vi "Process.vi"(8 "error in":errorcluster, 11 "main_UI":refnum<class "UI_main.lvclass">) -> (0 "error out":errorcluster, 3 "main_UI out":refnum<class "UI_main.lvclass">)   [LabVIEW 2016, in "UI_main.lvclass"]
doc: "---------------------------------------------------------------\nJKI State Machine Objects™\nhttp://jki.net/state-machine-objects/\nCopyright (C) 2005-2015, JKI <info@jki.net>\nALL RIGHTS RESERVED"
uses:
  UI_main.lvclass
  C:/Program Files (x86)/National Instruments/LabVIEW 2016/vi.lib/JKI/JKI SMO/SMO/SMO.lvclass
  <vilib>/JKI/JKI SMO/SMO/Typedefs/Parent Call--Enum.ctl
  SMO.Activity/SMO.Activity.lvclass
  <vilib>/JKI/JKI SMO/SMO/SMO.lvclass
  DAQ_config_UI/UI_DAQ_config.lvclass
  C:/user/patrick/hg/lockin.SMO/lvsrc/SMOs/SMO.Activity/SMO.Activity.lvclass
panel:
  in  "Shutdown":bool
  in  "config Lockin":bool
  in  "config DAQs":bool
  in  "show graphs":bool
  # "For instructions on how to use the JKI State Machine Objects, examples and video tutorials, visit:\nhttp://jki.net/state-machine-objects/\n\nJKI State Machine Objects™\nhttp://jki.net/state-machine-objects/\nCopyright (C) 2005-2015, JKI <info@jki.net>\nALL RIGHTS RESERVED"
  # "main UI: Always running?"
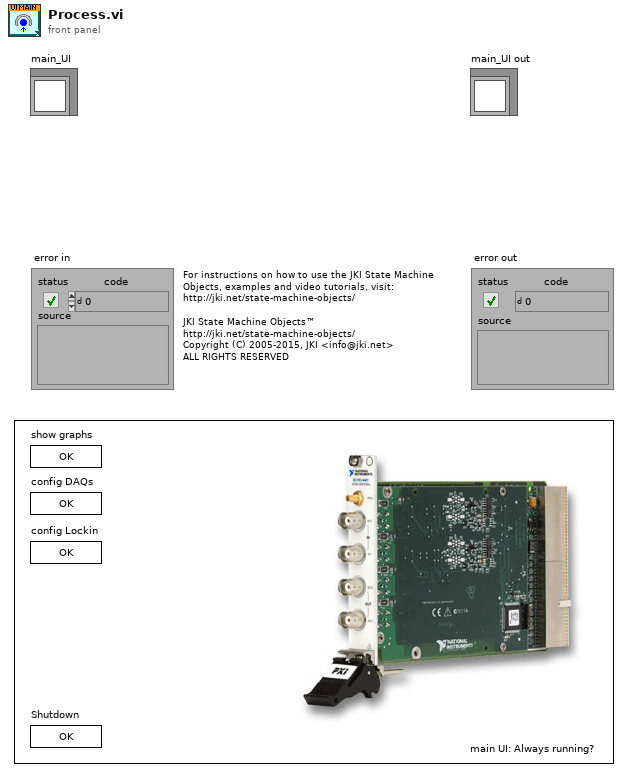
[diagram p1: front panel]
types:
  T1 = typedef "SMO.lvclass/Parent Call--Enum.ctl" = enum16{"Allows parent to run", "Does not request parent to run"}
  T2 = enum32{"invalid app kind", "Development System", "Run Time System", "Student Edition", "Embedded LabVIEW", "Evaluation", "Custom"}
  T3 = enum32{"Invalid", "Standard", "Closed", "Hidden", "Minimized", "Maximized"}
  T4 = enum32{"Bad", "Idle", "Run top level", "Running"}
  T5 = cluster{"Core":cluster{"Current VI Reference":refnum<vi>, "Close Panel on Exit?":bool, "error":errorcluster}, "Self Reference":refnum<class "UI_main.lvclass">, "Your string data":string, "SubUIs":refnum<class "SMO.Activity.lvclass">[]}
  T6 = cluster{"Current VI Reference":refnum<vi>, "Close Panel on Exit?":bool, "error":errorcluster}
  T7 = typedef "SMO.lvclass/Protected Events.ctl" = cluster{"StopProcesses":refnum<user-event>, "AbortProcesses":refnum<user-event>, "Config Changed":refnum<user-event>, "Dependency":refnum<user-event>}
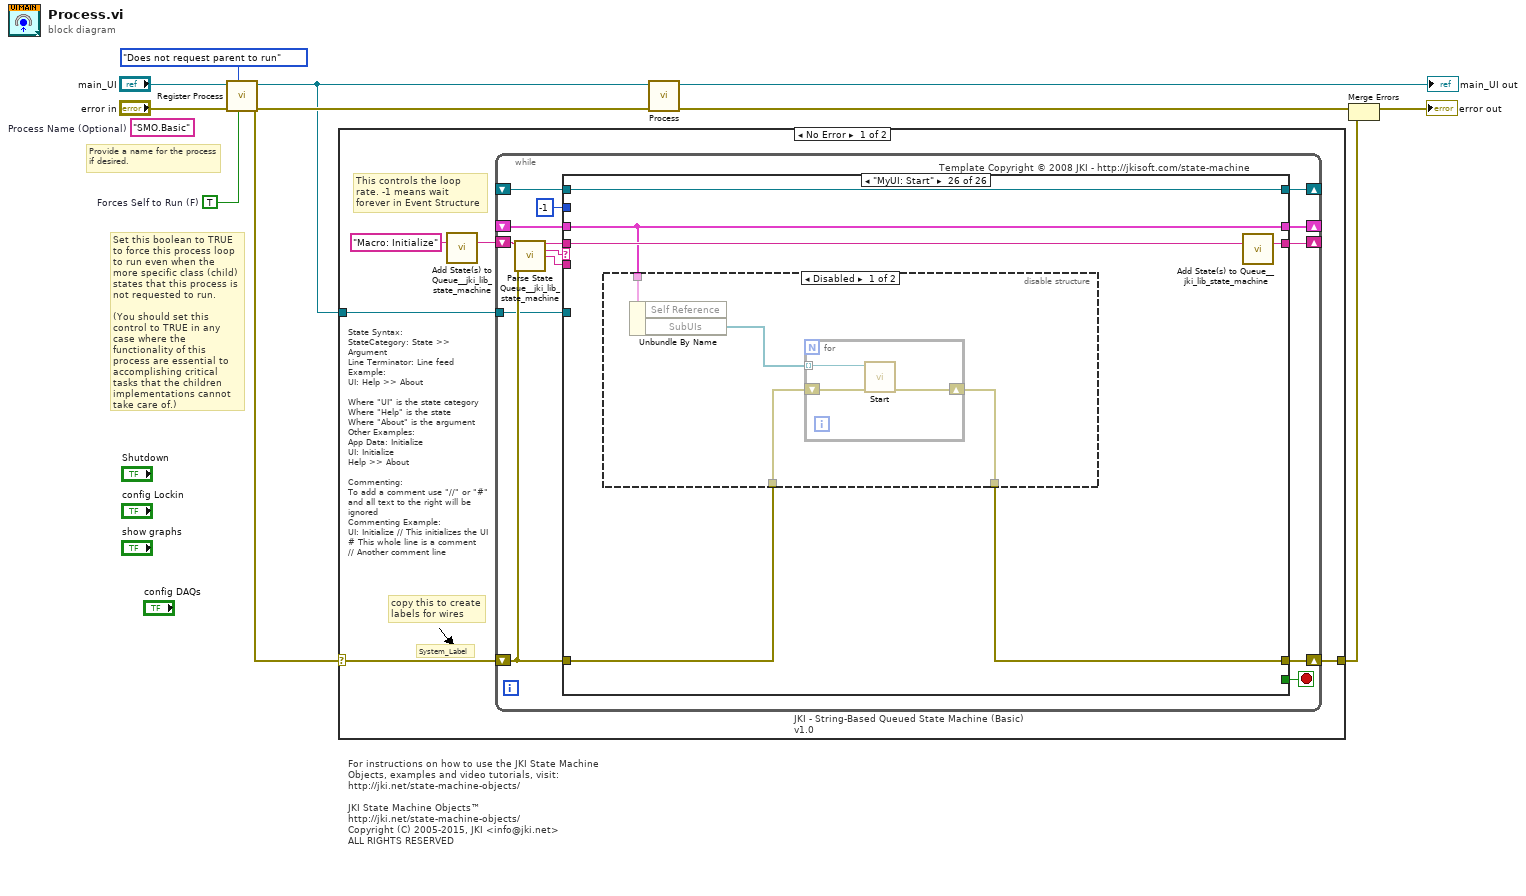
[diagram p0: block diagram]
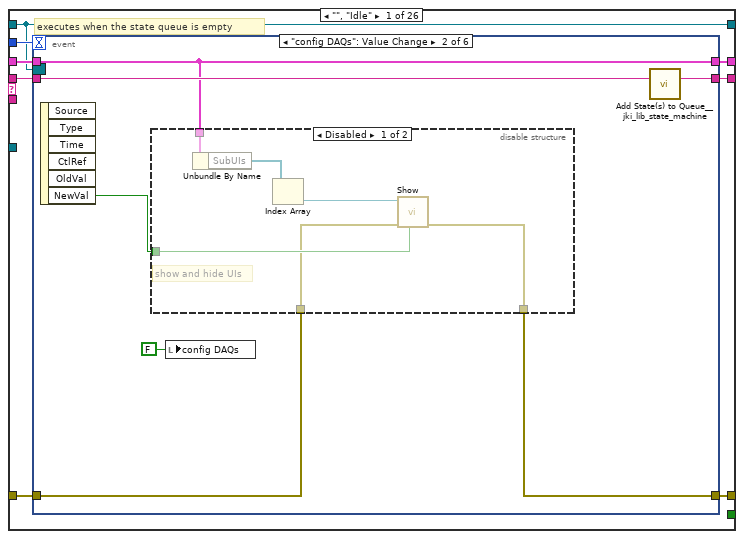
[diagram p2: hidden frame]
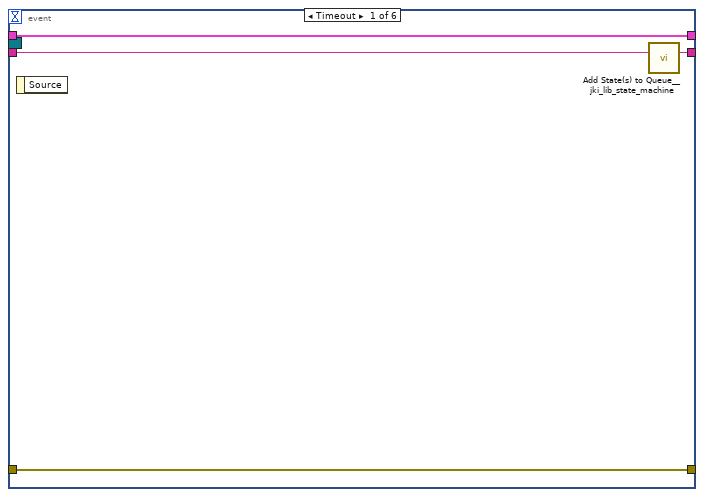
[diagram p3: hidden frame]
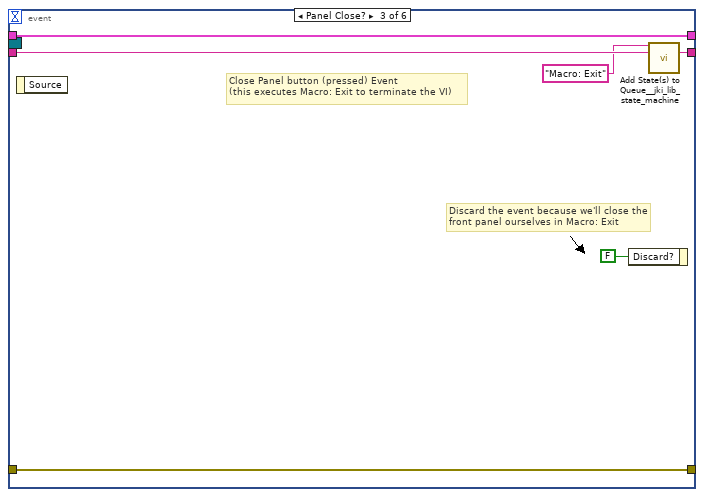
[diagram p5: hidden frame]
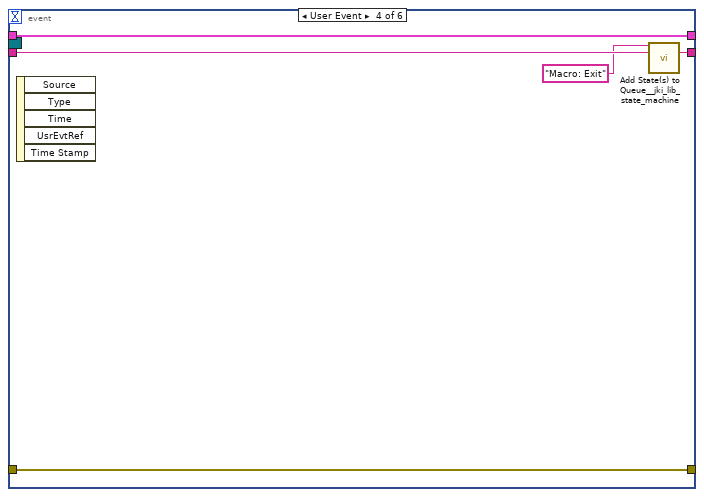
[diagram p6: hidden frame]
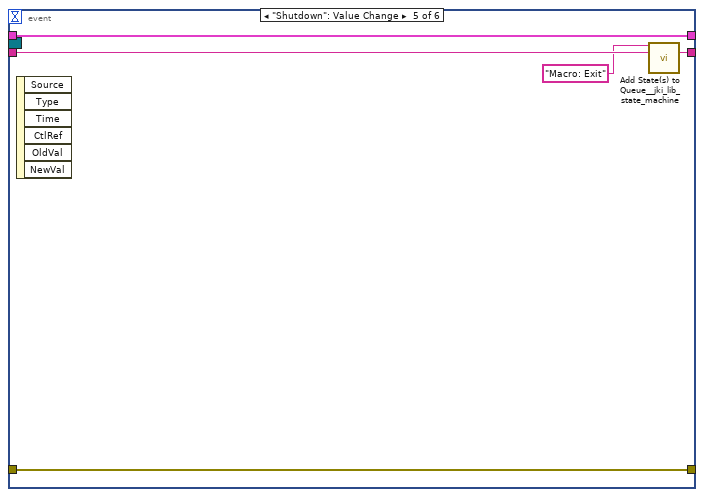
[diagram p7: hidden frame]
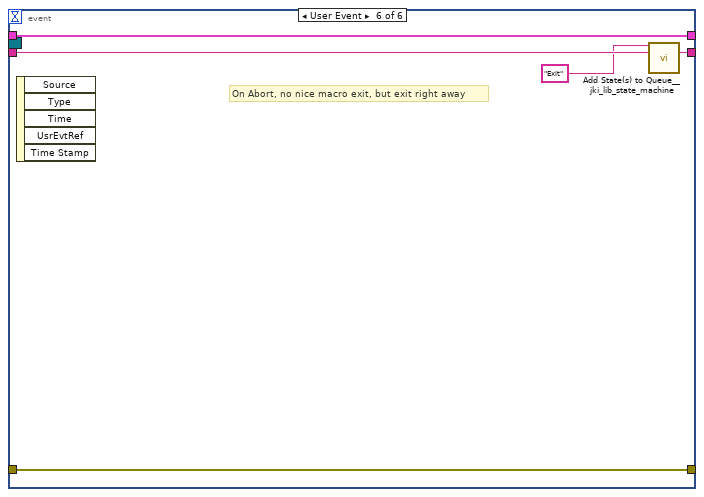
[diagram p8: hidden frame]
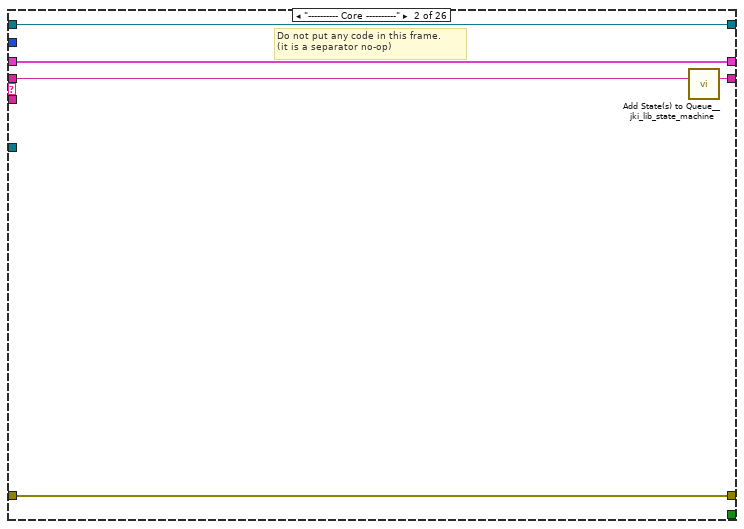
[diagram p9: hidden frame]
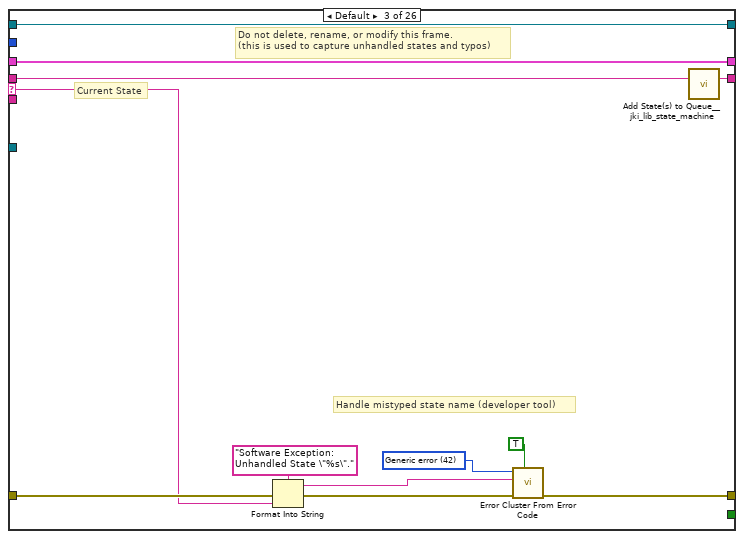
[diagram p10: hidden frame]
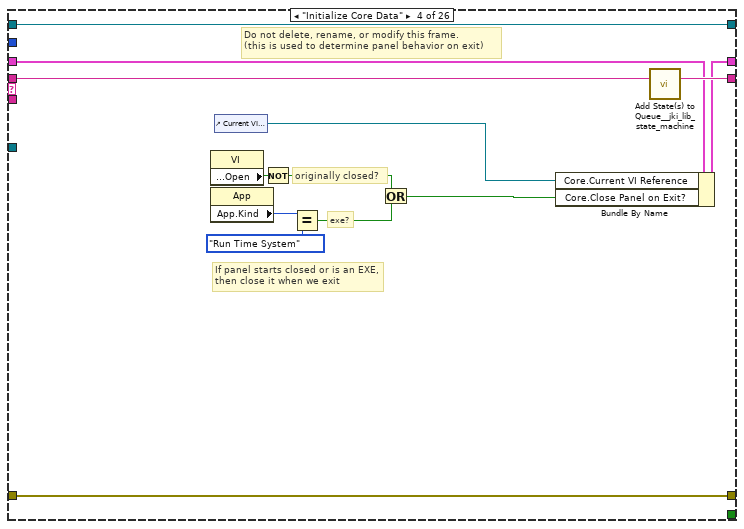
[diagram p11: hidden frame]
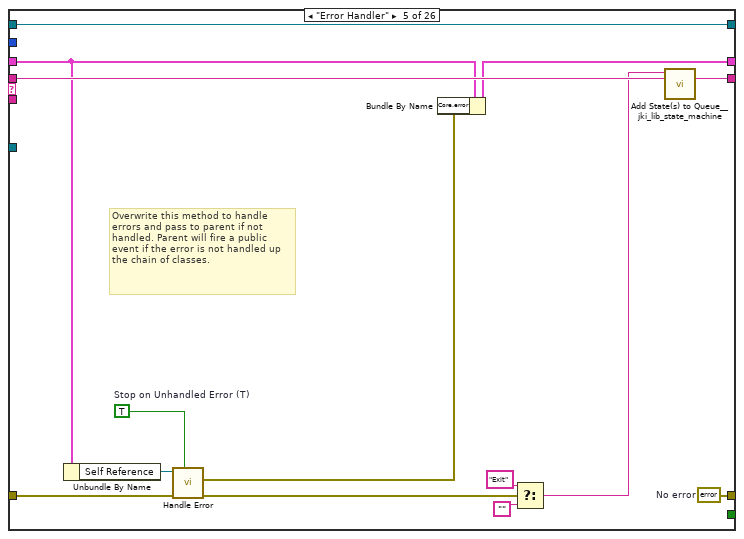
[diagram p12: hidden frame]
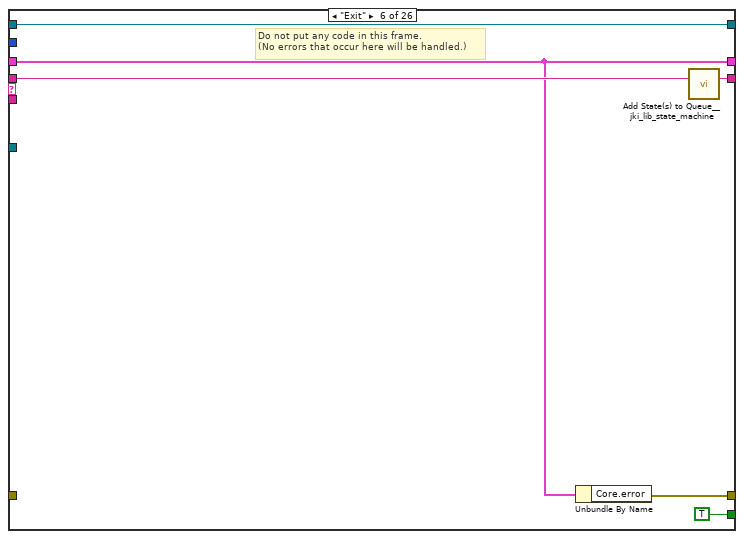
[diagram p13: hidden frame]
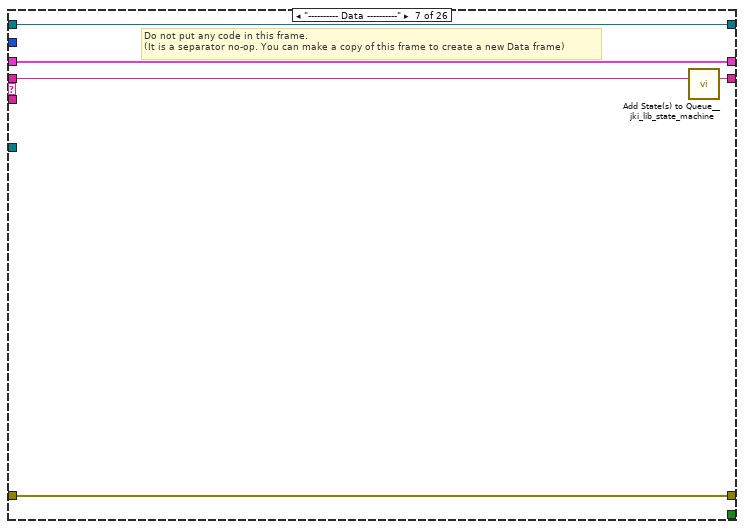
[diagram p14: hidden frame]
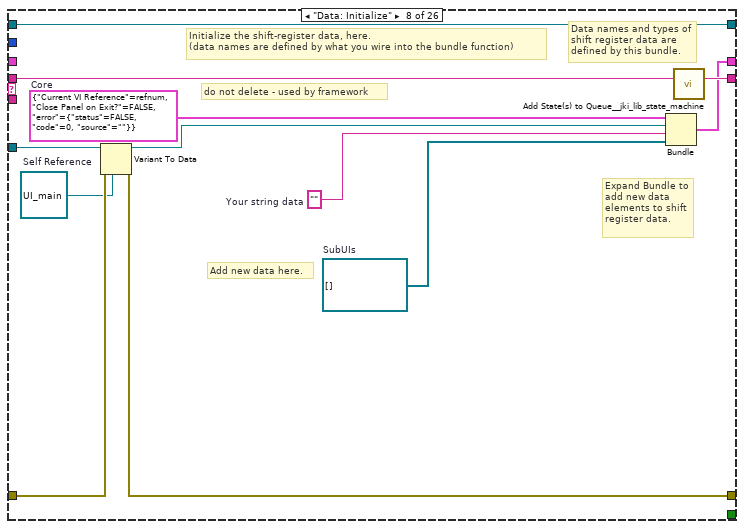
[diagram p15: hidden frame]
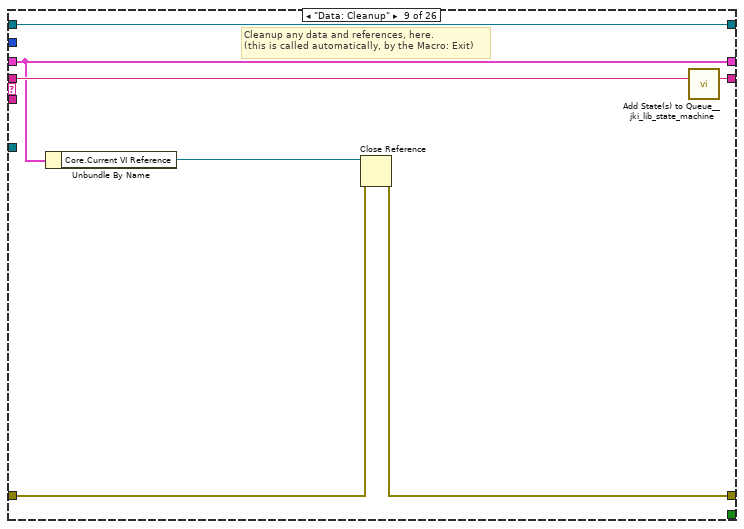
[diagram p16: hidden frame]
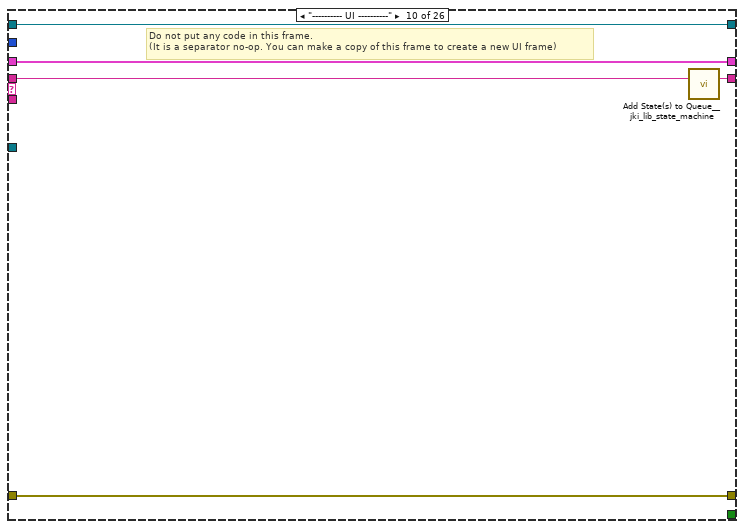
[diagram p17: hidden frame]
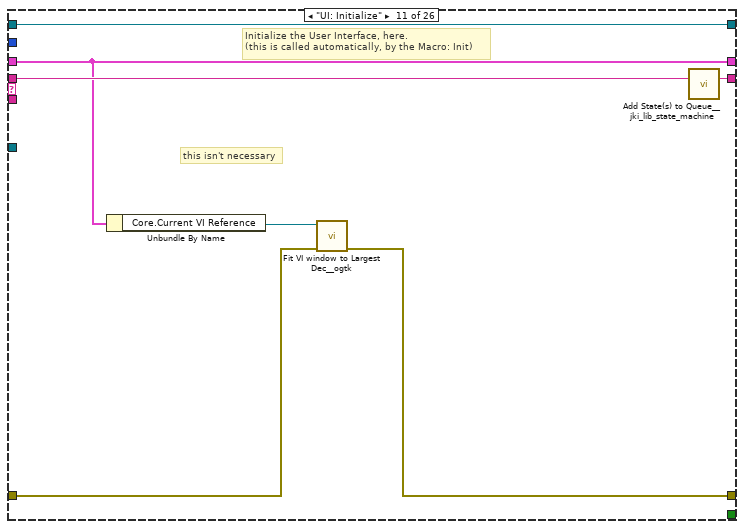
[diagram p18: hidden frame]
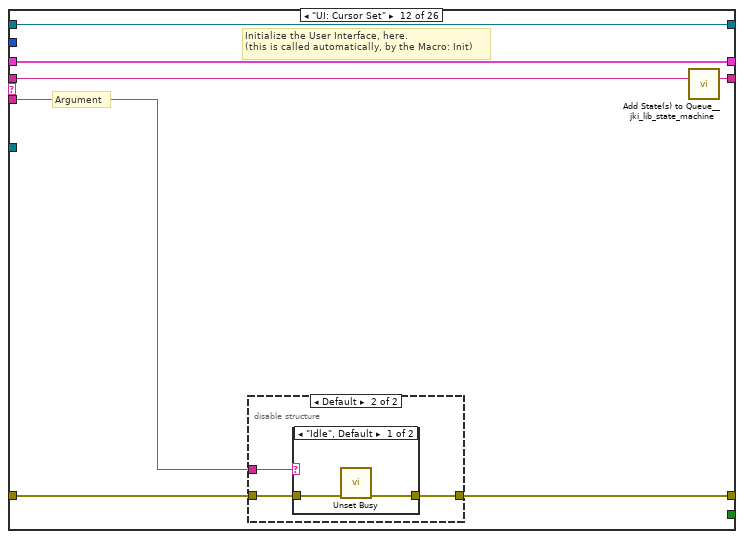
[diagram p19: hidden frame]
diagram:
  w1 = TRUE  # Forces Self to Run (F)
  (unwired) "SMO.Basic"  # Process Name (Optional)
  # "Provide a name for the process\nif desired."
  # "Set this boolean to TRUE to force this process loop to run even when the more specific class (child) states that this process is not requested to run.\n\n(You should set this control to TRUE in any case where the functionality of this process are essential to accomplishing critical tasks that the children implementations cannot take care of.)"
  # "For instructions on how to use the JKI State Machine Objects, examples and video tutorials, visit:\nhttp://jki.net/state-machine-objects/\n\nJKI State Machine Objects™\nhttp://jki.net/state-machine-objects/\nCopyright (C) 2005-2015, JKI <info@jki.net>\nALL RIGHTS RESERVED"
  n1 = call <vilib>:"Register Process.vi"("Forces Self to Run (F)"=w1, "Parent Call"=Parent_Call--Enum."Does not request parent to run", "error in (no error)"="error in", "SMO"="main_UI") -> ("error out"=w7:errorcluster, "SMO out"=w6:refnum<class "UI_main.lvclass">)  [unwired: 6 in]
  n2 = case shown="No Error" w7 {
    selector: w7 -> [w12 w354]
    tunnel: w6 -> [w13 _]
    tunnel: [w11 w354] -> w3
    frame No Error {
      # "State Syntax:\nStateCategory: State >> Argument\nLine Terminator: Line feed\nExample:\nUI: Help >> About\n\nWhere \"UI\" is the state category\nWhere \"Help\" is the state\nWhere \"About\" is the argument\nOther Examples:\nApp Data: Initialize\nUI: Initialize\nHelp >> About\n\nCommenting:\nTo add a comment use \"//\" or \"#\" and all text to the right will be ignored\nCommenting Example:\nUI: Initialize // This initializes the UI\n# This whole line is a comment\n// Another comment line"
      # "copy this to create labels for wires"
      # "This controls the loop rate. -1 means wait forever in Event Structure"
      # "System_Label"
      n3 = call <vilib>:"Add State(s) to Queue__jki_lib_state_machine.vi"("State(s) in (\"\")"="Macro: Initialize") -> ("States Out"=w15:string)  [unwired: 14 in]
      n4 = while "JKI - String-Based Queued State Machine (Basic) v1.0" {
        shift-right: [w22] -> _
        shift-left: _ -> [w21]
        shift-right: [w25] -> w11
        shift-left: w12 -> [w19]
        shift-right: [w24] -> _
        shift-left: w15 -> [w26]
        tunnel: w13 -> [w18]
        shift-right: [w17] -> _
        shift-left: _ -> [w16]
        stop <- w23 stop-if-true
        # "Template Copyright © 2008 JKI - http://jkisoft.com/state-machine"
        n5 = call <vilib>:"Parse State Queue__jki_lib_state_machine.vi"("State Queue"=w26, "Error In (no error)"=w19) -> ("Remaining States"=w28:string, "Current State"=w29:string, "Arguments"=w27:string)  [unwired: 11 in]
        n6 = case shown="\"MyUI: Start\"" w29 {
          selector: w29 -> [_ _ w82 _ _ _ _ _ _ _ _ _ _ _ _ _ _ _ _ _ _ _ _ _ _ _]
          tunnel: w28 -> [w37 w80 w86 w105 w119 w125 w130 w142 w149 w154 w161 w168 w186 w218 w232 w246 w251 w262 w267 w277 w283 w288 w295 w320 w333 w346]
          tunnel: w27 -> [_ _ _ _ _ _ _ _ _ _ _ w162 w181 _ _ _ _ _ _ _ _ _ _ _ _ _]
          tunnel: w21 -> [w35 w77 w84 w96 w113 w121 w127 _ w144 w151 w156 w166 w183 w215 w228 w237 w248 w259 w264 w275 w281 w286 w292 w317 w330 w343]
          tunnel: [w34 w78 w88 w102 w114 w120 w128 w137 w145 w152 w157 w163 w178 w216 w230 w244 w249 w253 w265 w270 w279 w284 w289 w315 w328 w341] -> w25
          tunnel: w19 -> [w33 w78 w87 w102 w115 _ w128 w138 w146 w152 w158 w164 w184 w216 w230 w244 w249 w254 w265 w271 w279 w284 w290 w316 w329 w342]
          tunnel: [w36 w79 w85 w104 w118 w124 w129 w141 w148 w153 w160 w167 w185 w217 w231 w245 w250 w261 w266 w276 w282 w287 w294 w319 w332 w345] -> w24
          tunnel: [_ _ _ _ _ TRUE _ _ _ _ _ _ _ _ _ _ _ _ _ _ _ _ _ _ _ _] -> w23
          tunnel: [w32 w77 w84 w103 w112 w121 w127 w140 w144 w151 w156 w166 w183 w215 w228 w237 w248 w259 w264 w275 w281 w286 w291 w317 w330 w343] -> w22
          tunnel: -1 ("Timeout") -> [w31 _ _ _ _ _ _ _ _ _ _ _ _ _ _ _ _ _ _ _ _ _ _ _ _ _]
          tunnel: w18 -> [_ _ _ _ _ _ _ w135 _ _ _ _ _ _ _ _ _ _ _ _ _ _ _ _ _ _]
          tunnel: [w30 w76 w81 w93 w117 w122 w126 w133 w143 w150 w159 w165 w180 w214 w229 w238 w247 w260 w263 w274 w280 w285 w293 w318 w331 w344] -> w17
          tunnel: w16 -> [w30 w76 w81 w93 w117 w122 w126 w133 w143 w150 w159 w165 w180 w214 w229 w238 w247 w260 w263 _ w280 w285 w293 w318 w331 w344]
          frame "", "Idle" {
            # "executes when the state queue is empty"
            n7 = event shown="[1] \"config DAQs\": Value Change" {
              selector: w30 -> [_ _ _ _ _ _]
              dyn-events: _ -> [_ _ _ _ _ _]
              timeout: w31 -> [_ _ _ _ _ _]
              tunnel: w37 -> [w41 w47 w60 w65 w70 w75]
              tunnel: [w40 w48 w59 w64 w69 w74] -> w36
              tunnel: w35 -> [w39 w46 w57 w62 w67 w72]
              tunnel: [w38 w44 w58 w63 w68 w73] -> w34
              tunnel: w33 -> [w38 w45 w58 w63 w68 w73]
              tunnel: [w39 w46 w57 w62 w67 w72] -> w32
              event Timeout {
                n8 = event-data() -> ()  [unwired: 1 in, 1 out]
                n9 = call <vilib>:"Add State(s) to Queue__jki_lib_state_machine.vi"("State(s) in (\"\")"=w41) -> ("States Out"=w40:string)  [unwired: 14 in]
              }
              event "config DAQs": Value Change {
                n10 = event-data() -> ("NewVal"=w43:bool)  [unwired: 1 in, 5 out]
                n11 = disable-structure shown="Disabled" {
                  disable-tunnel: w46 -> [w54 _]
                  disable-tunnel: w43 -> [w52 _]
                  disable-tunnel: w45 -> [w50 _]
                  disable-tunnel: [w49 _] -> w44
                  frame Disabled {
                    # "show and hide UIs"
                    n12 = Unbundle By Name(w54) -> ("SubUIs"=w53:refnum<class "SMO.Activity.lvclass">[])
                    n13 = Index Array(array=w53) -> (element=w51:refnum<class "SMO.Activity.lvclass">)  [unwired: 1 in]
                    n14 = call "Show.vi"("Force? (true)"=w52, "error in (no error)"=w50, "SMO.Activity"=w51) -> ("error out"=w49:errorcluster)  [unwired: 7 in, 1 out]
                  }
                  frame Enabled {
                  }
                }
                n15 = local write "config DAQs"(FALSE ("config DAQs")) -> ()
                n16 = call <vilib>:"Add State(s) to Queue__jki_lib_state_machine.vi"("State(s) in (\"\")"=w47) -> ("States Out"=w48:string)  [unwired: 14 in]
              }
              event Panel Close? {
                # "Discard the event because we'll close the front panel ourselves in Macro: Exit"
                # "Close Panel button (pressed) Event\n(this executes Macro: Exit to terminate the VI)"
                n17 = event-data() -> ()  [unwired: 1 in, 1 out]
                n18 = event-data("Discard?"=FALSE) -> ()  [unwired: 1 in, 1 out]
                n19 = call <vilib>:"Add State(s) to Queue__jki_lib_state_machine.vi"("State(s) in Front (\"\")"="Macro: Exit", "State(s) in (\"\")"=w60) -> ("States Out"=w59:string)  [unwired: 13 in]
              }
              event User Event {
                n20 = event-data() -> ()  [unwired: 1 in, 5 out]
                n21 = call <vilib>:"Add State(s) to Queue__jki_lib_state_machine.vi"("State(s) in Front (\"\")"="Macro: Exit", "State(s) in (\"\")"=w65) -> ("States Out"=w64:string)  [unwired: 13 in]
              }
              event "Shutdown": Value Change {
                n22 = event-data() -> ()  [unwired: 1 in, 6 out]
                n23 = call <vilib>:"Add State(s) to Queue__jki_lib_state_machine.vi"("State(s) in Front (\"\")"="Macro: Exit", "State(s) in (\"\")"=w70) -> ("States Out"=w69:string)  [unwired: 13 in]
              }
              event User Event {
                # "On Abort, no nice macro exit, but exit right away"
                n24 = event-data() -> ()  [unwired: 1 in, 5 out]
                n25 = call <vilib>:"Add State(s) to Queue__jki_lib_state_machine.vi"("State(s) in Front (\"\")"="Exit", "State(s) in (\"\")"=w75) -> ("States Out"=w74:string)  [unwired: 13 in]
              }
            }
          }
          frame "---------- Core ----------" {
            # "Do not put any code in this frame.\n(it is a separator no-op)"
            n26 = call <vilib>:"Add State(s) to Queue__jki_lib_state_machine.vi"("State(s) in (\"\")"=w80) -> ("States Out"=w79:string)  [unwired: 14 in]
          }
          frame Default {
            w91 = 42 items=["No error", "Argument error", "Memory is full", "Out of zone", "End of file", "File already open", "Generic file I/O error", "File not found", "File permission error", "Disk is full", "Duplicate path", "Too many files open", "System feature not enabled", "Resource file not found", "Cannot add resource", "Resource not found", "Image not found", "Image memory error", "Pen does not exist", "Config type invalid", "Config token not found", "Config parse error", "Config memory error", "Bad external code format", "Bad external code offset", "External code not present", "Null window", "Destroy window error", "Null menu", "Print aborted", "Bad print record", "Print driver error", "Windows error during printing", "Memory error during printing", "Print dialog error", "Generic print error", "Invalid device refnum", "Device not found", "Device parameter error", "Device unit error", "Cannot open device", "Device call aborted", "Generic error", "Cancelled by user", "Object ID too low", "Object ID too high", "Object not in heap", "Unknown heap", "Unknown object (invalid DefProc)", "Unknown object (DefProc not in table)", "Message out of range", "Invalid (null) method", "Unknown message", "Manager call not supported", "Bad address", "Network operation in progress", "Network operation timed out", "Connection is busy", "Network attribute not supported", "Network error", "Address in use", "System out of memory", "Connection aborted", "Connection refused", "Not connected", "Already connected", "Connection closed", "Initialization error (interapplication manager)", "Bad occurrence", "Wait on unbound occurrence handler", "Occurrence queue overflow", "Datalog type conflict", "Unused", "Unrecognized type (interapplication manager)", "Memory corrupt", "Failed to make temporary DLL", "Old CIN version", "Drag socket not found", "Failed to load drop-object", "Failed to register OLE object", "Failed to release OLE object", "Format specifier type mismatch", "Unknown format specifier", "Too few format specifiers", "Too many format specifiers", "Scan failed", "Newer CIN version", "Error converting to variant", "Runtime menu error", "Password tampered", "Variant attribute not found", "Incompatible variant data type", "Event data is not available", "Event Store is not present", "Occurrence is not found", "Event Queue is not created", "Event info is not available", "Refnum passed is NULL", "Error retrieving Class GUID", "Error retrieving CoClass GUID", "Error retrieving TypeLib GUID.", "Bad built application magic bytes.", "Specific driver is different from the specific driver associated with the Logical Name.", "There is no session opened to the class driver.", "Max Error", "MAX - Error with config objects", "MAX - Error loading configuration", "MAX - Group not supported"]
            # "Current State"
            # "Do not delete, rename, or modify this frame.\n(this is used to capture unhandled states and typos)"
            # "Handle mistyped state name (developer tool)"
            n27 = Format Into String(format string="Software Exception: Unhandled State \"%s\"." ("message"), error in=w87, w82) -> (resulting string=w90:string, error out=w89:errorcluster)  [unwired: 1 in]
            n28 = call <vilib>:"Error Cluster From Error Code.vi"("show call chain? (False)"=TRUE, "error in (no error)"=w89, "error message (\"\")"=w90, "error code (0)"=w91) -> ("error out"=w88:errorcluster)  [unwired: 5 in]
            n29 = call <vilib>:"Add State(s) to Queue__jki_lib_state_machine.vi"("State(s) in (\"\")"=w86) -> ("States Out"=w85:string)  [unwired: 14 in]
          }
          frame "Initialize Core Data" {
            # "Do not delete, rename, or modify this frame.\n(this is used to determine panel behavior on exit)"
            # "originally closed?"
            # "exe?"
            # "If panel starts closed or is an EXE, then close it when we exit"
            n30 = property class="VI"() -> ("Front Panel.Open"=w101:bool)  [unwired: 2 in, 2 out]
            n31 = property class="App"() -> ("App.Kind"=w100:T2)  [unwired: 2 in, 2 out]
            n32 = control-ref of="Current VI Reference"() -> (w94:refnum<vi>)
            n33 = Not(x=w101) -> (.not. x?=w98:bool)
            n34 = Equal?(x=w100, y=T2."Run Time System" ("Application:Kind")) -> (x = y?=w97:bool)
            n35 = Or(x=w98, y=w97) -> (x .or. y?=w95:bool)
            n36 = Bundle By Name(cluster=w96, "Core.Current VI Reference"=w94, "Core.Close Panel on Exit?"=w95) -> (w103:T5)
            n37 = call <vilib>:"Add State(s) to Queue__jki_lib_state_machine.vi"("State(s) in (\"\")"=w105) -> ("States Out"=w104:string)  [unwired: 14 in]
          }
          frame "Error Handler" {
            w106 = TRUE  # Stop on Unhandled Error (T)
            w114 = errorcluster {"status"=FALSE, "code"=0, "source"=""}  # No error
            # "Overwrite this method to handle errors and pass to parent if not handled. Parent will fire a public event if the error is not handled up the chain of classes."
            n38 = Unbundle By Name(w113) -> ("Self Reference"=w116:refnum<class "UI_main.lvclass">)
            n39 = call-dynamic "Handle Error.vi"("Stop on Unhandled Error (T)"=w106, "error in"=w115, "SMO"=w116) -> ("handling error"=w107:errorcluster, "Unhandled error"=w110:errorcluster)  [unwired: 6 in, 1 out]
            n40 = Bundle By Name(cluster=w113, "Core.error"=w110) -> (w112:T5)
            n41 = Select(t="Exit", s=w107, f="") -> (s? t:f=w111:string)
            n42 = call <vilib>:"Add State(s) to Queue__jki_lib_state_machine.vi"("State(s) in Front (\"\")"=w111, "State(s) in (\"\")"=w119) -> ("States Out"=w118:string)  [unwired: 13 in]
          }
          frame "Exit" {
            # "Do not put any code in this frame.\n(No errors that occur here will be handled.)"
            n43 = Unbundle By Name(w121) -> ("Core.error"=w120:errorcluster)
            n44 = call <vilib>:"Add State(s) to Queue__jki_lib_state_machine.vi"("State(s) in (\"\")"=w125) -> ("States Out"=w124:string)  [unwired: 14 in]
          }
          frame "---------- Data ----------" {
            # "Do not put any code in this frame.\n(It is a separator no-op. You can make a copy of this frame to create a new Data frame)"
            n45 = call <vilib>:"Add State(s) to Queue__jki_lib_state_machine.vi"("State(s) in (\"\")"=w130) -> ("States Out"=w129:string)  [unwired: 14 in]
          }
          frame "Data: Initialize" {
            w131 = refnum<class "SMO.Activity.lvclass">[] []  # SubUIs
            w132 = T6 {"Current VI Reference"=refnum, "Close Panel on Exit?"=FALSE, "error"={"status"=FALSE, "code"=0, "source"=""}}  # Core
            w136 = refnum<class "UI_main.lvclass"> refnum  # Self Reference
            w139 = ""  # Your string data
            # "do not delete - used by framework"
            # "Expand Bundle to add new data elements to shift register data."
            # "Add new data here."
            # "Data names and types of shift register data are defined by this bundle."
            # "Initialize the shift-register data, here.\n(data names are defined by what you wire into the bundle function)"
            n46 = Variant To Data(error in=w138, type=w136, Variant=w135) -> (data=w134:refnum<class "UI_main.lvclass">, error out=w137:errorcluster)
            n47 = Bundle("Core"=w132, "Self Reference"=w134, "Your string data"=w139, "SubUIs"=w131) -> (w140:T5)  [unwired: 1 in]
            n48 = call <vilib>:"Add State(s) to Queue__jki_lib_state_machine.vi"("State(s) in (\"\")"=w142) -> ("States Out"=w141:string)  [unwired: 14 in]
          }
          frame "Data: Cleanup" {
            # "Cleanup any data and references, here.\n(this is called automatically, by the Macro: Exit)"
            n49 = Unbundle By Name(w144) -> ("Core.Current VI Reference"=w147:refnum<vi>)
            n50 = Close Reference(reference=w147, error in (no error)=w146) -> (error out=w145:errorcluster)
            n51 = call <vilib>:"Add State(s) to Queue__jki_lib_state_machine.vi"("State(s) in (\"\")"=w149) -> ("States Out"=w148:string)  [unwired: 14 in]
          }
          frame "---------- UI ----------" {
            # "Do not put any code in this frame.\n(It is a separator no-op. You can make a copy of this frame to create a new UI frame)"
            n52 = call <vilib>:"Add State(s) to Queue__jki_lib_state_machine.vi"("State(s) in (\"\")"=w154) -> ("States Out"=w153:string)  [unwired: 14 in]
          }
          frame "UI: Initialize" {
            # "this isn't necessary"
            # "Initialize the User Interface, here.\n(this is called automatically, by the Macro: Init)"
            n53 = Unbundle By Name(w156) -> ("Core.Current VI Reference"=w155:refnum<vi>)
            n54 = call <userlib>:"Fit VI window to Largest Dec__ogtk.vi"("error in (no error)"=w158, "VI Ref (calling VI)"=w155) -> ("error out"=w157:errorcluster)  [unwired: 4 in, 1 out]
            n55 = call <vilib>:"Add State(s) to Queue__jki_lib_state_machine.vi"("State(s) in (\"\")"=w161) -> ("States Out"=w160:string)  [unwired: 14 in]
          }
          frame "UI: Cursor Set" {
            # "Argument"
            # "Initialize the User Interface, here.\n(this is called automatically, by the Macro: Init)"
            n56 = disable-structure shown="Default" {
              disable-tunnel: w164 -> [w169 w172]
              disable-tunnel: [w169 w171] -> w163
              disable-tunnel: w162 -> [_ w170]
              frame condition #0 {
              }
              frame condition #1 (active) {
                n57 = case shown="\"Idle\", Default" w170 {
                  tunnel: w172 -> [w174 w176]
                  tunnel: [w173 w175] -> w171
                  frame "Idle", Default {
                    n58 = call <vilib>:"Unset Busy.vi"("error in (no error)"=w174) -> ("error out"=w173:errorcluster)  [unwired: 10 in]
                  }
                  frame "Busy" {
                    n59 = call <vilib>:"Set Busy.vi"("error in (no error)"=w176) -> ("error out"=w175:errorcluster)  [unwired: 9 in, 1 out]
                  }
                }
              }
            }
            n60 = call <vilib>:"Add State(s) to Queue__jki_lib_state_machine.vi"("State(s) in (\"\")"=w168) -> ("States Out"=w167:string)  [unwired: 14 in]
          }
          frame "UI: Front Panel State" {
            # "Argument"
            # "Set Front Panel Open or Closed\n(Usage: \"UI: Front Panel State >> Open|Close\")"
            n61 = Unbundle By Name(w183) -> ("Core.Current VI Reference"=w182:refnum<vi>)
            n62 = disable-structure shown="Default" {
              disable-tunnel: w184 -> [w190 w213]
              disable-tunnel: [w189 w213] -> w179
              disable-tunnel: w182 -> [w188 _]
              disable-tunnel: w181 -> [w187 _]
              frame condition #0 (active) {
                n63 = case shown="\"Close\"" w187 {
                  tunnel: w190 -> [w194 w207]
                  tunnel: [w196 w208] -> w189
                  tunnel: w188 -> [w195 w205]
                  frame "Open", Default {
                    n64 = property class="VI"(reference=w195, error in=w194) -> (reference out=w192:refnum<vi>, error out=w193:errorcluster, "FP.State"=w191:T3)
                    n65 = case shown="\"Closed\"" w191 {
                      tunnel: [w199 w202] -> w196
                      tunnel: w193 -> [w198 w202]
                      tunnel: w192 -> [w197 _]
                      frame "Closed" {
                        n66 = invoke class="VI" method="FP.Open"(reference=w197, error in=w198, "Activate"=TRUE, "State"=T3."Standard") -> (error out=w199:errorcluster)  [unwired: 1 in, 4 out]
                      }
                      frame Default {
                      }
                    }
                  }
                  frame "Close" {
                    n67 = property class="VI"(reference=w205, error in=w207) -> (reference out=w204:refnum<vi>, error out=w206:errorcluster, "FP.State"=w203:T3)
                    n68 = case shown="Default" w203 {
                      tunnel: [w209 w212] -> w208
                      tunnel: w206 -> [w209 w211]
                      tunnel: w204 -> [_ w210]
                      frame "Invalid", "Closed" {
                      }
                      frame Default {
                        n69 = invoke class="VI" method="FP.Close"(reference=w210, error in=w211) -> (error out=w212:errorcluster)  [unwired: 1 in, 2 out]
                      }
                    }
                  }
                }
              }
              frame condition #1 {
              }
            }
            n70 = call <userlib>:"Wait (ms)__ogtk.vi"("error in (no error)"=w179, "milliseconds to wait"=u32 5000) -> ("error out"=w178:errorcluster)  [unwired: 8 in, 1 out]
            n71 = call <vilib>:"Add State(s) to Queue__jki_lib_state_machine.vi"("State(s) in (\"\")"=w186) -> ("States Out"=w185:string)  [unwired: 14 in]
          }
          frame "---------- Macro ----------" {
            # "Do not put any code in this frame.\n(It is a separator no-op. You can make a copy of this frame to create a new Macro frame)"
            n72 = call <vilib>:"Add State(s) to Queue__jki_lib_state_machine.vi"("State(s) in (\"\")"=w218) -> ("States Out"=w217:string)  [unwired: 14 in]
          }
          frame "Macro: Initialize" {
            w223 = "UI: Initialize\nUI: Front Panel State >> Open\nMyUI: Create\nMyUI: Start"  # UI: Initialize UI: Front Panel State >> Open MyUI: Create MyUI: Start
            w219 = "Process: Sync"
            # "Initialization Macro\n(This is called once, when the VI starts)"
            n73 = control-ref of="This VI"() -> (w221:refnum<vi>)
            n74 = property class="VI"(reference=w221) -> ("Exec.State"=w220:T4)  [unwired: 1 in, 2 out]
            n75 = Equal?(x=w220, y=T4."Run top level") -> (x = y?=w226:bool)
            n76 = Select(t=w219, s=w226, f="") -> ()  [unwired: 1 out]
            n77 = call <vilib>:"Add State(s) to Queue__jki_lib_state_machine.vi"("State(s) in Front (\"\")"="Data: Initialize\nInitialize Core Data\nEvents: Register", "State(s) in (\"\")"=w219, "State(s) at Back (\"\")"=w223) -> ("States Out"=w222:string)  [unwired: 12 in]
            n78 = call <vilib>:"Add State(s) to Queue__jki_lib_state_machine.vi"("State(s) in Front (\"\")"=w222, "State(s) in (\"\")"=w232) -> ("States Out"=w231:string)  [unwired: 13 in]
          }
          frame "Macro: Exit" {
            # "Exit Macro\n(This is called once, when the VI exits)"
            n79 = Unbundle By Name(w237) -> ("Core.Close Panel on Exit?"=w243:bool)
            n80 = Select(t="UI: Front Panel State >> Close", s=w243, f="") -> (s? t:f=w240:string)
            n81 = call <vilib>:"Add State(s) to Queue__jki_lib_state_machine.vi"("State(s) in Front (\"\")"="MyUI: Destroy\nData: Cleanup\nEvents: Unregister", "State(s) in (\"\")"="Process: Sync", "State(s) at Back (\"\")"="Exit") -> ("States Out"=w234:string)  [unwired: 12 in]
            n82 = call <vilib>:"Add State(s) to Queue__jki_lib_state_machine.vi"("State(s) in (\"\")"=w240, "State(s) at Back (\"\")"=w234) -> ("States Out"=w239:string)  [unwired: 13 in]
            n83 = call <vilib>:"Add State(s) to Queue__jki_lib_state_machine.vi"("State(s) in Front (\"\")"=w239, "State(s) in (\"\")"=w246) -> ("States Out"=w245:string)  [unwired: 13 in]
          }
          frame "---------- Process ----------" {
            # "Template Separator\n(You can make a copy of, or modify, this frame)"
            n84 = call <vilib>:"Add State(s) to Queue__jki_lib_state_machine.vi"("State(s) in (\"\")"=w251) -> ("States Out"=w250:string)  [unwired: 14 in]
          }
          frame "Process: Sync" {
            n85 = Unbundle By Name(w259) -> ("Self Reference"=w255:refnum<class "UI_main.lvclass">)
            n86 = call <vilib>:"WaitOnProcessSync.vi"("error in (no error)"=w254, "SMO"=w255) -> ("error out"=w253:errorcluster, "Don't run?"=w258:bool)  [unwired: 7 in, 1 out]
            n87 = Select(t="Data: Cleanup\nEvents: Unregister\nExit", s=w258, f="") -> (s? t:f=w252:string)
            n88 = call <vilib>:"Add State(s) to Queue__jki_lib_state_machine.vi"("State(s) in Front (\"\")"=w252, "State(s) in (\"\")"=w262) -> ("States Out"=w261:string)  [unwired: 13 in]
          }
          frame "---------- Events ----------" {
            # "Template Separator\n(You can make a copy of, or modify, this frame)"
            n89 = call <vilib>:"Add State(s) to Queue__jki_lib_state_machine.vi"("State(s) in (\"\")"=w267) -> ("States Out"=w266:string)  [unwired: 14 in]
          }
          frame "Events: Register" {
            # "Expand to add\nmore events"
            n90 = Unbundle By Name(w275) -> ("Self Reference"=w272:refnum<class "UI_main.lvclass">)
            n91 = call <vilib>:"GetProtectedEvents.vi"("SMO"=w272) -> ("error out"=w268:errorcluster, "SMO Protected Events"=w273:T7)  [unwired: 8 in, 1 out]
            n92 = register-events(w273) -> (reference out=w274:refnum<event-registration>, error out=w269:errorcluster)  [unwired: 2 in]
            n93 = Merge Errors(w271, w269, w268) -> (w270:errorcluster)
            n94 = call <vilib>:"Add State(s) to Queue__jki_lib_state_machine.vi"("State(s) in (\"\")"=w277) -> ("States Out"=w276:string)  [unwired: 14 in]
          }
          frame "Events: Unregister" {
            n95 = Unregister For Events(event registration refnum=w280, error in=w279) -> (error out=w278:errorcluster)
            n96 = call <vilib>:"Clear Errors.vi"("error in (no error)"=w278) -> ()  [unwired: 5 in, 2 out]
            n97 = call <vilib>:"Add State(s) to Queue__jki_lib_state_machine.vi"("State(s) in (\"\")"=w283) -> ("States Out"=w282:string)  [unwired: 14 in]
          }
          frame "---------- Action ----------" {
            n98 = call <vilib>:"Add State(s) to Queue__jki_lib_state_machine.vi"("State(s) in (\"\")"=w288) -> ("States Out"=w287:string)  [unwired: 14 in]
          }
          frame "MyUI: Create" {
            n99 = disable-structure shown="Disabled" {
              disable-tunnel: w292 -> [w307 _]
              disable-tunnel: [w306 _] -> w291
              disable-tunnel: w290 -> [w305 _]
              disable-tunnel: [w296 _] -> w289
              frame Disabled {
                # "placeholder for other UIs\neg, UI_DSP_config, UI_scope, etc"
                # "create UI_DAQ_config"
                n100 = Unbundle By Name(w307) -> ("Self Reference"=w304:refnum<class "UI_main.lvclass">)
                n101 = Unbundle By Name(w304) -> ("lockin"=w303:refnum<class "lockin.lvclass">)
                n102 = call "Create UI_DAQ_config.vi"("error in (no error)"=w305, "lockin"=w303) -> ("error out"=w301:errorcluster, "DAQ_config_UI out"=w300:refnum<class "UI_DAQ_config.lvclass">)  [unwired: 8 in]
                n103 = disable-structure shown="Disabled" {
                  disable-tunnel: [w314 _] -> w302
                  disable-tunnel: w301 -> [w313 _]
                  disable-tunnel: [w312 _] -> w299
                  frame Disabled {
                    n104 = call "Create UI_DAQ_config.vi"("error in (no error)"=w313) -> ("error out"=w312:errorcluster, "DAQ_config_UI out"=w314:refnum<class "UI_DAQ_config.lvclass">)  [unwired: 9 in]
                  }
                  frame Enabled {
                  }
                }
                n105 = Build Array(w300, w302) -> (w298:refnum<class "UI_DAQ_config.lvclass">[])
                n106 = for {
                  tunnel: w298 -> [w310] mode=indexing
                  tunnel: [w309] -> w297 mode=indexing
                  shift-right: [w308] -> w296
                  shift-left: w299 -> [w311]
                  n107 = call <vilib>:"Start.vi"("error in (no error)"=w311, "SMO"=w310) -> ("error out"=w308:errorcluster, "SMO out"=w309:refnum<class "UI_DAQ_config.lvclass">)  [unwired: 8 in]
                }
                n108 = Bundle By Name(cluster=w307, "Self Reference"=w304, "SubUIs"=w297) -> (w306:T5)
              }
              frame Enabled {
              }
            }
            n109 = call <vilib>:"Add State(s) to Queue__jki_lib_state_machine.vi"("State(s) in (\"\")"=w295) -> ("States Out"=w294:string)  [unwired: 14 in]
          }
          frame "MyUI: Destroy" {
            n110 = disable-structure shown="Disabled" {
              disable-tunnel: w317 -> [w323 _]
              disable-tunnel: w316 -> [w322 _]
              disable-tunnel: [w321 _] -> w315
              frame Disabled {
                n111 = Unbundle By Name(w323) -> ("SubUIs"=w324:refnum<class "SMO.Activity.lvclass">[])  [unwired: 1 out]
                n112 = for {
                  tunnel: w324 -> [w327] mode=indexing
                  shift-right: [w325] -> w321
                  shift-left: w322 -> [w326]
                  n113 = call <vilib>:"Destroy.vi"("error in (no error)"=w326, "SMO"=w327) -> ("error out"=w325:errorcluster)  [unwired: 9 in]
                }
              }
              frame Enabled {
              }
            }
            n114 = call <vilib>:"Add State(s) to Queue__jki_lib_state_machine.vi"("State(s) in (\"\")"=w320) -> ("States Out"=w319:string)  [unwired: 14 in]
          }
          frame "MyUI: Stop" {
            n115 = disable-structure shown="Disabled" {
              disable-tunnel: w330 -> [w337 _]
              disable-tunnel: w329 -> [w336 _]
              disable-tunnel: [w335 _] -> w328
              frame Disabled {
                n116 = Unbundle By Name(w337) -> ("SubUIs"=w334:refnum<class "SMO.Activity.lvclass">[])  [unwired: 1 out]
                n117 = for {
                  tunnel: w334 -> [w338] mode=indexing
                  shift-right: [w339] -> w335
                  shift-left: w336 -> [w340]
                  n118 = call <vilib>:"Stop.vi"("error in (no error)"=w340, "SMO"=w338) -> ("error out"=w339:errorcluster)  [unwired: 8 in, 1 out]
                }
              }
              frame Enabled {
              }
            }
            n119 = call <vilib>:"Add State(s) to Queue__jki_lib_state_machine.vi"("State(s) in (\"\")"=w333) -> ("States Out"=w332:string)  [unwired: 14 in]
          }
          frame "MyUI: Start" {
            n120 = disable-structure shown="Disabled" {
              disable-tunnel: w343 -> [w350 _]
              disable-tunnel: w342 -> [w349 _]
              disable-tunnel: [w348 _] -> w341
              frame Disabled {
                n121 = Unbundle By Name(w350) -> ("SubUIs"=w347:refnum<class "SMO.Activity.lvclass">[])  [unwired: 1 out]
                n122 = for {
                  tunnel: w347 -> [w351] mode=indexing
                  shift-right: [w352] -> w348
                  shift-left: w349 -> [w353]
                  n123 = call <vilib>:"Start.vi"("error in (no error)"=w353, "SMO"=w351) -> ("error out"=w352:errorcluster)  [unwired: 8 in, 1 out]
                }
              }
              frame Enabled {
              }
            }
            n124 = call <vilib>:"Add State(s) to Queue__jki_lib_state_machine.vi"("State(s) in (\"\")"=w346) -> ("States Out"=w345:string)  [unwired: 14 in]
          }
        }
      }
    }
    frame Error {
    }
  }
  n125 = call-parent "Process.vi"("error in"=w7, "SMO"=w6) -> ("error out"=w4:errorcluster, "SMO out"=→"main_UI out":refnum<class "UI_main.lvclass">)  [unwired: 8 in]
  n126 = Merge Errors(w4, w3) -> (→"error out":errorcluster)
